vi "motorisedmirrors_coMD.vi"() -> ()   [LabVIEW 2012]
doc: "SciScan 1.2 160622"
uses:
  GFG/GFGstringGet.vi
  <vilib>/Instr/_visa.llb/VISA Configure Serial Port (Instr).vi
  GFG/GFG library.lvlib
panel:
  out "error out":errorcluster
  in  "lock":bool
  in  "SCANHEAD":bool
  in  "MDU":bool
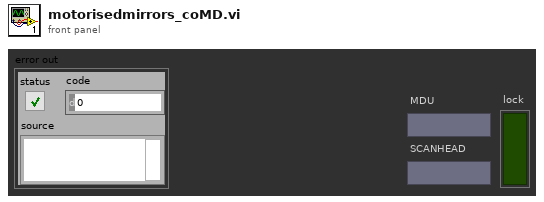
[diagram p1: front panel]
types:
  T1 = enum32{"Invalid", "Standard", "Closed", "Hidden", "Minimized", "Maximized"}
  T2 = enum8{"Enabled", "Disabled", "Disabled and Grayed Out"}
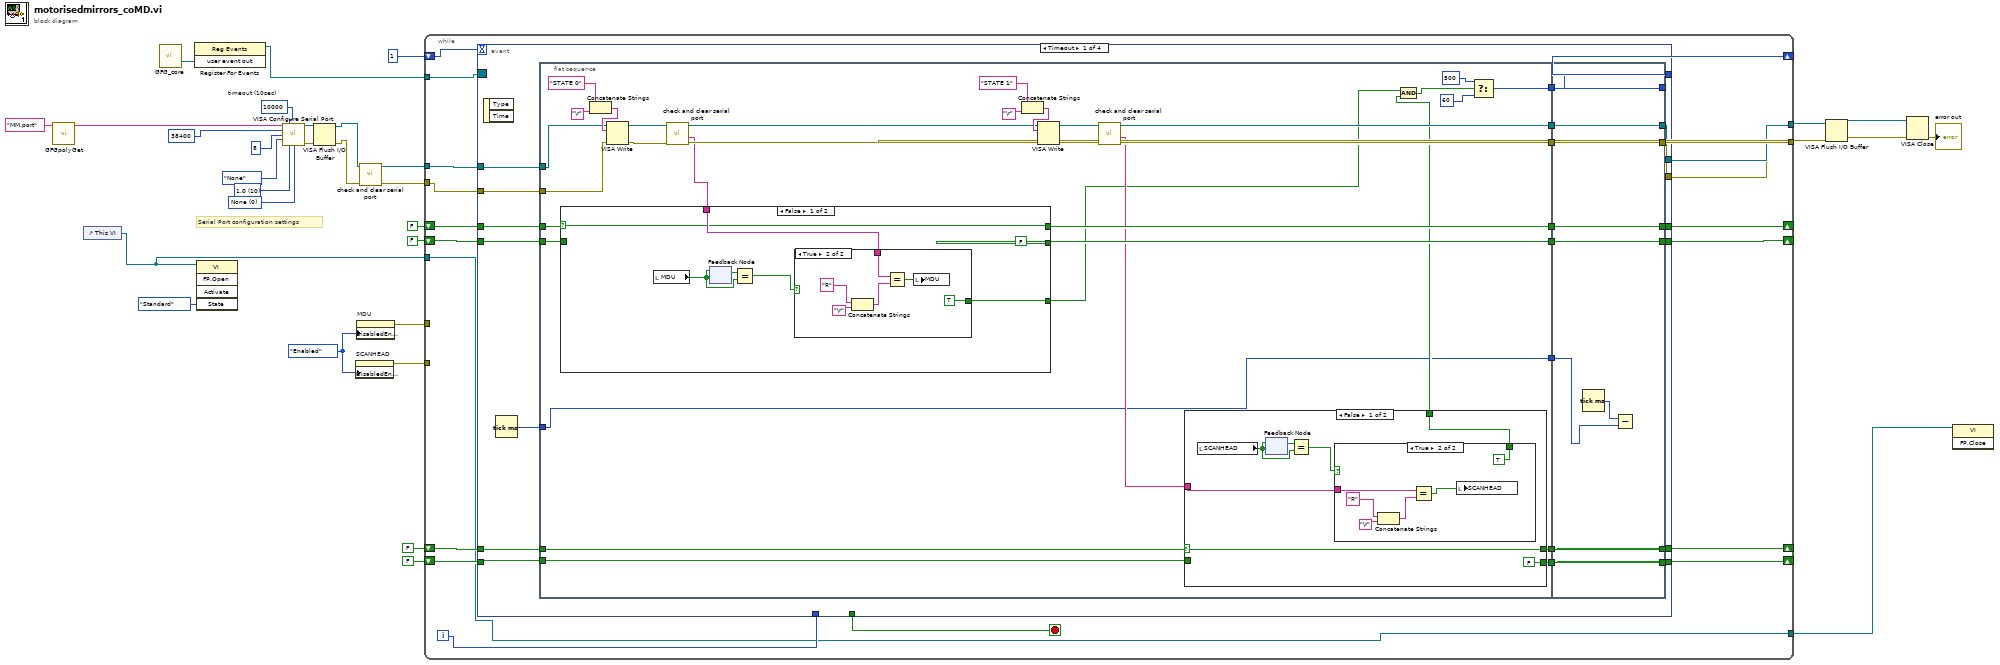
[diagram p0: block diagram]
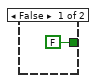
[diagram p2: hidden frame]
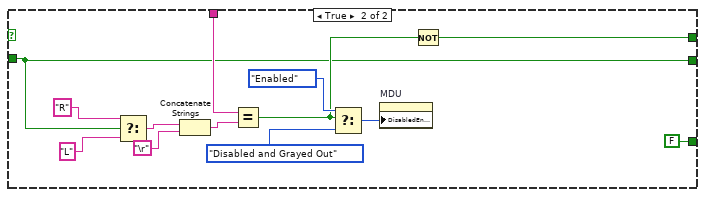
[diagram p3: hidden frame]
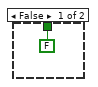
[diagram p4: hidden frame]
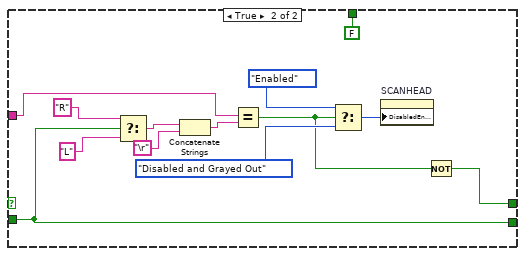
[diagram p5: hidden frame]
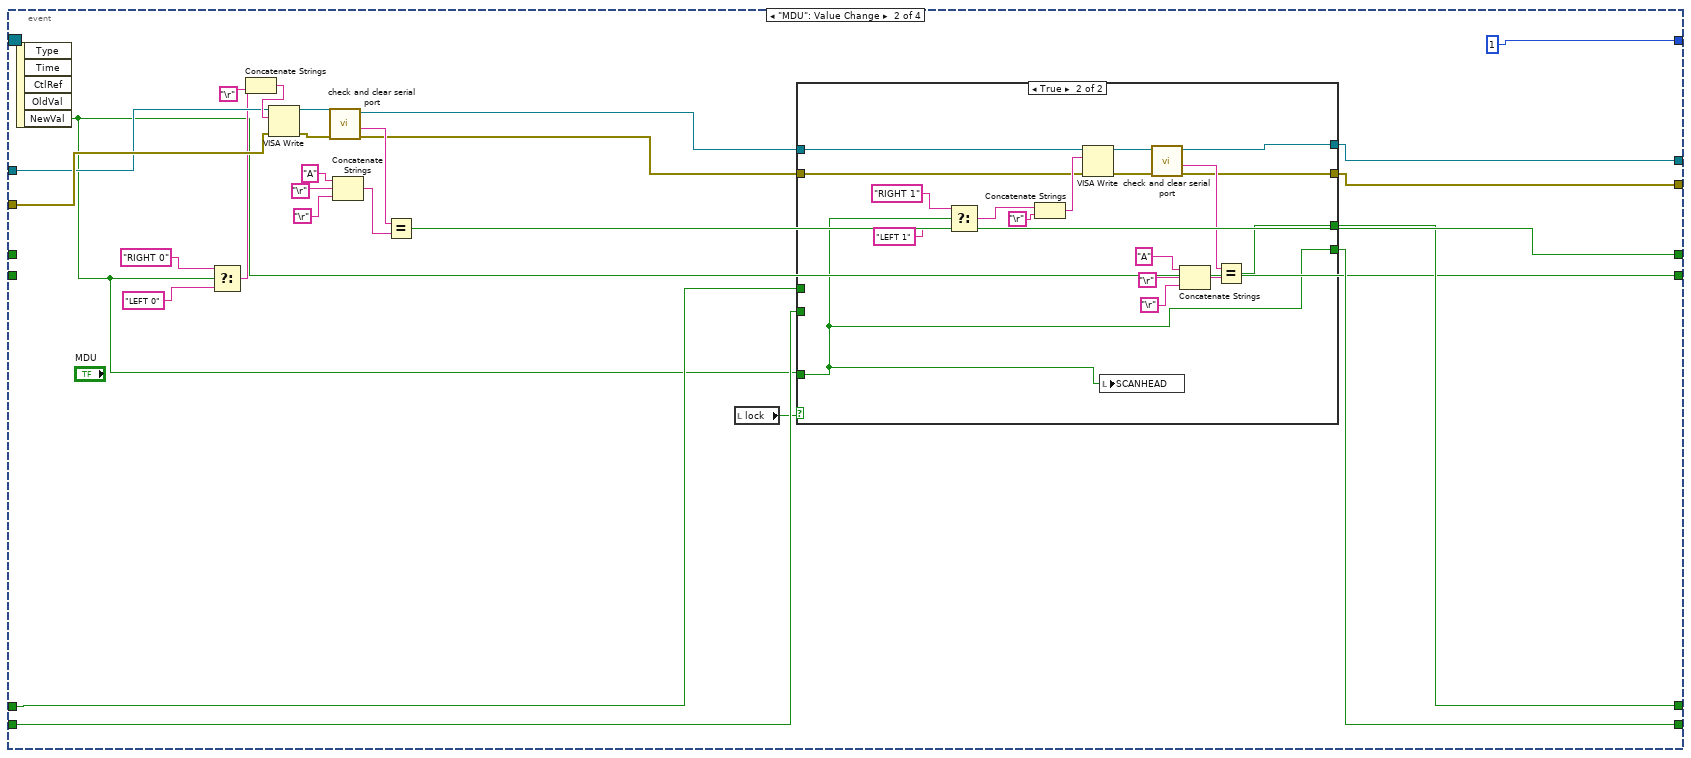
[diagram p6: hidden frame]
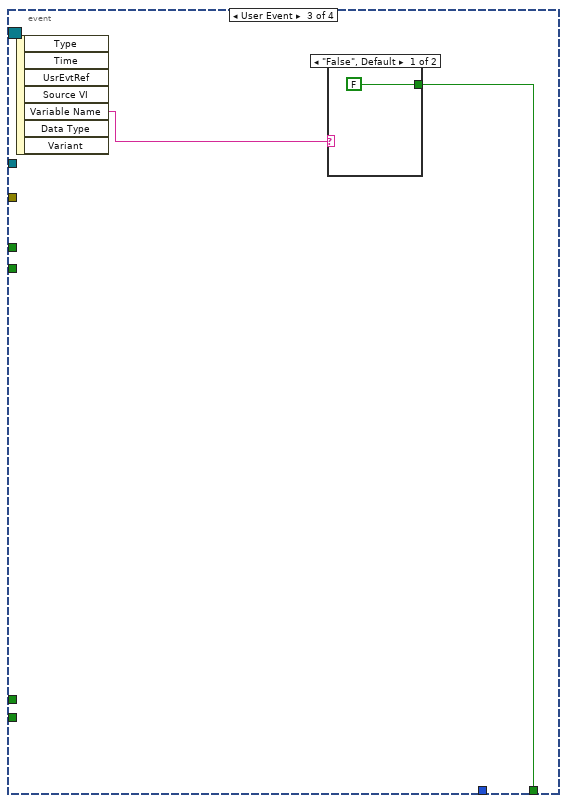
[diagram p8: hidden frame]
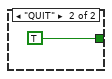
[diagram p9: hidden frame]
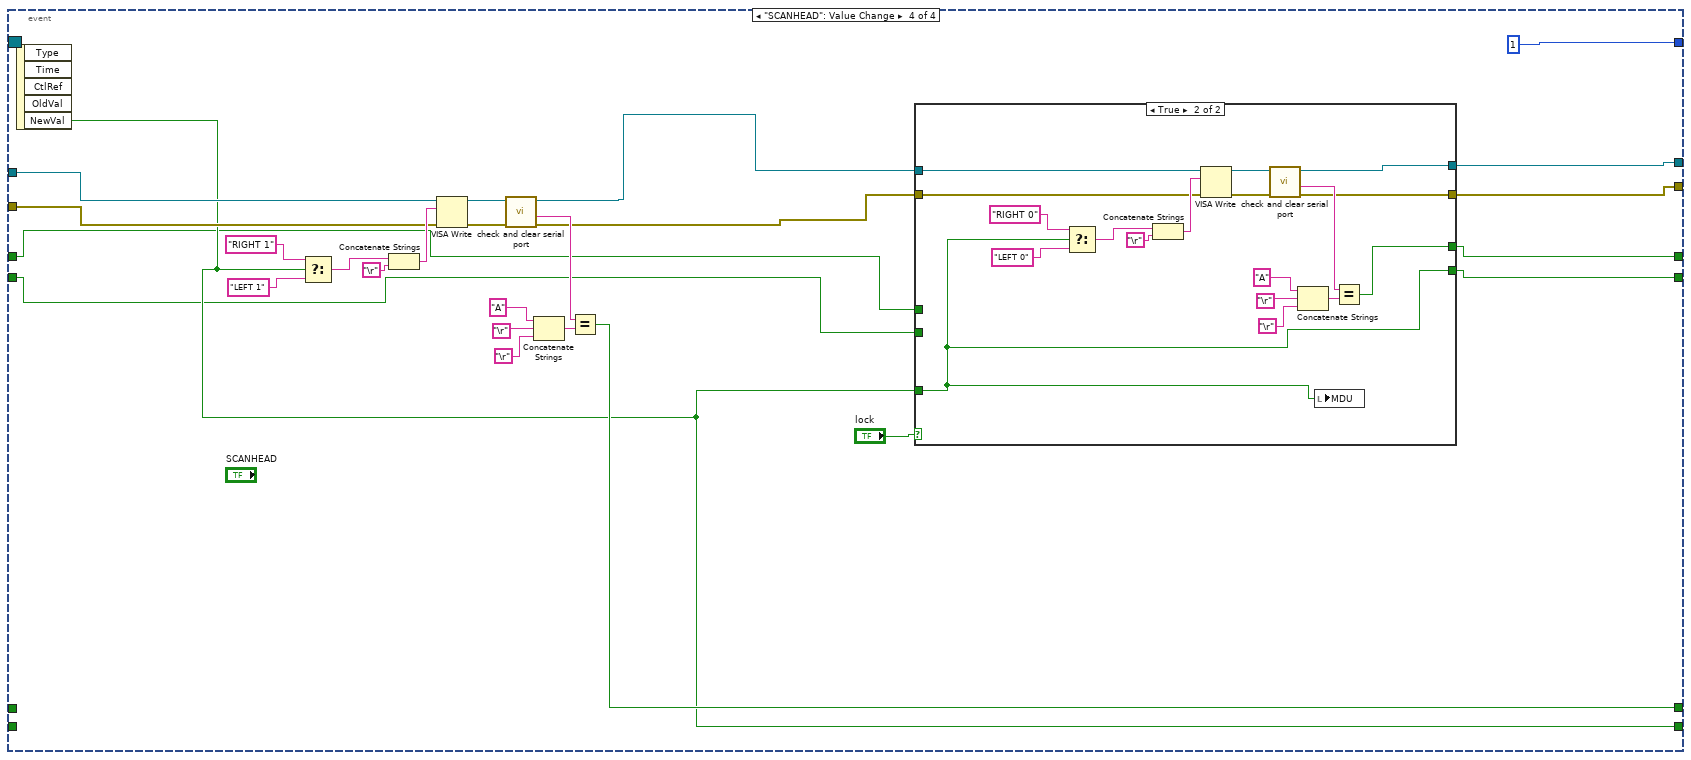
[diagram p10: hidden frame]
diagram:
  w11 = T2."Enabled" ("Disabled")
  w29 = u16 0 items=["None", "XON/XOFF", "RTS/CTS", "XON/XOFF & RTS/CTS", "DTR/DSR", "XON/XOFF & DTR/DSR"] ("flow control (0:none)")
  w28 = u16 10 items=["1.0"=10, "1.5"=15, "2.0"=20] ("stop bits (10: 1 bit)")
  w25 = u32 10000  # timeout (10sec)
  # "Serial Port configuration settings"
  n1 = call-poly "GFGpolyGet.vi"("Variable Name in"="MM.port") -> ("String"=w4:string)  [unwired: 9 in, 1 out]
  n2 = control-ref of="This VI"() -> (w2:refnum<vi>)
  n3 = call "GFG_core.vi"() -> ("user event out"=w8:refnum<user-event>)  [unwired: 13 in, 6 out]
  n4 = register-events(w8) -> (reference out=w7:refnum<event-registration>)  [unwired: 2 in, 1 out]
  n5 = invoke class="VI" method="FP.Open"(reference=w2, "State"=T1."Standard") -> ()  [unwired: 3 in, 5 out]
  n6 = call-poly "VISA Configure Serial Port"("VISA resource name"=w4, "timeout (10sec)"=w25, "baud rate (9600)"=38400, "data bits (8)"=u16 8, "parity (0:none)"=enum16{"None", "Odd", "Even", "Mark", "Space"}."None", "stop bits (10: 1 bit)"=w28, "flow control (0:none)"=w29) -> ("VISA resource name out"=w30:refnum<visa-resource-name>, "error out"=w31:errorcluster)  [unwired: 7 in]
  n7 = VISA Flush I/O Buffer(VISA resource name=w30, error in (no error)=w31) -> (VISA resource name out=w23:refnum<visa-resource-name>, error out=w24:errorcluster)  [unwired: 1 in]
  n8 = property on="SCANHEAD" class="Bool (strict)"("DisabledEnum"=w11) -> (error out=w9:errorcluster)  [unwired: 2 in, 1 out]
  n9 = property on="MDU" class="Bool (strict)"("DisabledEnum"=w11) -> (error out=w10:errorcluster)  [unwired: 2 in, 1 out]
  n10 = call "check and clear serial port.vi"("error in (no error)"=w24, "VISA resource name in"=w23) -> ("error out"=w21:errorcluster, "VISA resource name out"=w22:refnum<visa-resource-name>)  [unwired: 6 in, 2 out]
  n11 = while {
    tunnel: [w50] -> w16
    tunnel: [w49] -> w20
    tunnel: w22 -> [w48]
    tunnel: w21 -> [w47]
    shift-right: [w45] -> _
    shift-left: FALSE -> [w38]
    shift-right: [w43] -> _
    shift-left: 1 -> [w46]
    shift-right: [w42] -> _
    shift-left: FALSE ("MDU") -> [w37]
    shift-right: [w41] -> _
    shift-left: FALSE ("SCANHEAD") -> [w39]
    shift-right: [w44] -> _
    shift-left: FALSE -> [w40]
    tunnel: w10 -> [_]
    tunnel: w9 -> [_]
    tunnel: w7 -> [w35]
    tunnel: w2 -> [w33]
    tunnel: [w33] -> w1
    i -> [w36]
    stop <- w34 stop-if-true
    n12 = event shown="[0] Timeout" {
      selector: w35 -> [_ _ _ _]
      dyn-events: _ -> [_ _ _ _]
      timeout: w46 -> [_ _ _ _]
      tunnel: [w69 w169 _ w229] -> w50
      tunnel: [w70 w176 _ w227] -> w49
      tunnel: w48 -> [w72 w187 _ w240]
      tunnel: w47 -> [w71 w188 _ w241]
      tunnel: [w67 w180 _ w221] -> w45
      tunnel: [w68 w172 _ w231] -> w44
      tunnel: [w64 1 _ 1] -> w43
      tunnel: [w62 w170 _ w222] -> w42
      tunnel: [w60 w173 _ w225] -> w41
      tunnel: w40 -> [w66 w175 _ _]
      tunnel: w39 -> [w61 w174 _ _]
      tunnel: w38 -> [w65 _ _ w224]
      tunnel: w37 -> [w63 _ _ w223]
      tunnel: w36 -> [_ _ _ _]
      tunnel: [_ _ w217 _] -> w34
      event Timeout {
        n13 = event-data() -> ()  [unwired: 1 in, 2 out]
        n14 = Tick Count (ms)() -> (millisecond timer value=w59:u32)
        n15 = flat-sequence {
          tunnel: w72 -> [w103]
          tunnel: w71 -> [w102]
          tunnel: w66 -> [w87]
          tunnel: w65 -> [w86]
          tunnel: w63 -> [w82]
          tunnel: w61 -> [w80]
          tunnel: w59 -> [w73]
          tunnel: [w91] -> w58
          tunnel: [w90] -> w57
          tunnel: [w89] -> w56
          tunnel: [w88] -> w55
          tunnel: [w85] -> w54
          tunnel: [w81] -> w53
          tunnel: [w79] -> w52
          tunnel: [w73] -> w51
          tunnel: [w162] -> w60
          tunnel: [w163] -> w62
          tunnel: [w164] -> w64
          tunnel: [w165] -> w67
          tunnel: [w166] -> w68
          tunnel: [w167] -> w69
          tunnel: [w168] -> w70
          tunnel: w58 -> [w168]
          tunnel: w57 -> [w167]
          tunnel: w56 -> [w166]
          tunnel: w55 -> [w165]
          tunnel: w54 -> [w164]
          tunnel: w53 -> [w163]
          tunnel: w52 -> [w162]
          tunnel: w51 -> [w160]
          frame #0 {
            n16 = Concatenate Strings("STATE 0" ("string"), "\r") -> (w105:string)
            n17 = VISA Write(VISA resource name=w103, write buffer=w105, error in (no error)=w102) -> (VISA resource name out=w95:refnum<visa-resource-name>, error out=w101:errorcluster)  [unwired: 1 out]
            n18 = call "check and clear serial port.vi"("error in (no error)"=w101, "VISA resource name in"=w95) -> ("error out"=w94:errorcluster, "read buffer"=w77:string, "VISA resource name out"=w93:refnum<visa-resource-name>)  [unwired: 6 in, 1 out]
            n19 = case shown="False" w86 {
              selector: w86 -> [w111 _]
              tunnel: w77 -> [w112 w127]
              tunnel: [w111 w123] -> w88
              tunnel: w82 -> [_ w121]
              tunnel: [FALSE ("MDU") w121] -> w81
              tunnel: [w109 FALSE ("SCANHEAD")] -> w76
              frame False {
                n20 = local read "MDU"() -> (w108:bool)
                n21 = feedback #1() -> (w107:bool)  [unwired: 1 in]
                n22 = feedback-in #1(w108) -> ()
                n23 = Equal?(x=w107, y=w108) -> (x = y?=w106:bool)
                n24 = case shown="True" w106 {
                  tunnel: w112 -> [_ w116]
                  tunnel: [FALSE ("SCANHEAD") TRUE ("SCANHEAD")] -> w109
                  frame False {
                  }
                  frame True {
                    n25 = Concatenate Strings("R" ("y"), "\r") -> (w119:string)
                    n26 = Equal?(x=w116, y=w119) -> (x = y?=w115:bool)
                    n27 = local write "MDU"(w115) -> ()
                  }
                }
              }
              frame True {
                n28 = Select(t="R" ("string"), s=w121, f="L" ("string")) -> (s? t:f=w129:string)
                n29 = Concatenate Strings(w129, "\r") -> (w132:string)
                n30 = Equal?(x=w127, y=w132) -> (x = y?=w124:bool)
                n31 = Select(t=T2."Enabled" ("Disabled"), s=w124, f=T2."Disabled and Grayed Out" ("Disabled")) -> (s? t:f=w122:T2)
                n32 = property on="MDU" class="Bool (strict)"("DisabledEnum"=w122) -> ()  [unwired: 2 in, 2 out]
                n33 = Not(x=w124) -> (.not. x?=w123:bool)
              }
            }
            n34 = Concatenate Strings("STATE 1" ("string"), "\r") -> (w96:string)
            n35 = VISA Write(VISA resource name=w93, write buffer=w96, error in (no error)=w94) -> (VISA resource name out=w92:refnum<visa-resource-name>, error out=w98:errorcluster)  [unwired: 1 out]
            n36 = call "check and clear serial port.vi"("error in (no error)"=w98, "VISA resource name in"=w92) -> ("error out"=w91:errorcluster, "read buffer"=w78:string, "VISA resource name out"=w90:refnum<visa-resource-name>)  [unwired: 6 in, 1 out]
            n37 = case shown="False" w87 {
              selector: w87 -> [w138 _]
              tunnel: w78 -> [w139 w154]
              tunnel: [w138 w149] -> w89
              tunnel: w80 -> [_ w148]
              tunnel: [FALSE ("SCANHEAD") w148] -> w79
              tunnel: [w136 FALSE ("SCANHEAD")] -> w75
              frame False {
                n38 = local read "SCANHEAD"() -> (w134:bool)
                n39 = feedback #2() -> (w135:bool)  [unwired: 1 in]
                n40 = feedback-in #2(w134) -> ()
                n41 = Equal?(x=w135, y=w134) -> (x = y?=w133:bool)
                n42 = case shown="True" w133 {
                  tunnel: w139 -> [_ w143]
                  tunnel: [FALSE ("SCANHEAD") TRUE ("SCANHEAD")] -> w136
                  frame False {
                  }
                  frame True {
                    n43 = Concatenate Strings("R" ("y"), "\r") -> (w146:string)
                    n44 = Equal?(x=w143, y=w146) -> (x = y?=w142:bool)
                    n45 = local write "SCANHEAD"(w142) -> ()
                  }
                }
              }
              frame True {
                n46 = Select(t="R" ("string"), s=w148, f="L" ("string")) -> (s? t:f=w156:string)
                n47 = Concatenate Strings(w156, "\r") -> (w159:string)
                n48 = Equal?(x=w154, y=w159) -> (x = y?=w150:bool)
                n49 = Select(t=T2."Enabled" ("Disabled"), s=w150, f=T2."Disabled and Grayed Out" ("Disabled")) -> (s? t:f=w151:T2)
                n50 = property on="SCANHEAD" class="Bool (strict)"("DisabledEnum"=w151) -> ()  [unwired: 2 in, 2 out]
                n51 = Not(x=w150) -> (.not. x?=w149:bool)
              }
            }
            n52 = And(x=w76, y=w75) -> (x .and. y?=w74:bool)
            n53 = Select(t=500, s=w74, f=60) -> (s? t:f=w85:i32)
          }
          frame #1 {
            n54 = Tick Count (ms)() -> (millisecond timer value=w161:u32)
            n55 = Subtract(x=w161, y=w160) -> ()  [unwired: 1 out]
          }
        }
      }
      event "MDU": Value Change {
        n56 = event-data() -> ("NewVal"=w170:bool)  [unwired: 1 in, 4 out]
        n57 = Select(t="RIGHT 0" ("write buffer"), s=w170, f="LEFT 0" ("write buffer 2")) -> (s? t:f=w186:string)
        n58 = Concatenate Strings(w186, "\r") -> (w192:string)
        n59 = VISA Write(VISA resource name=w187, write buffer=w192, error in (no error)=w188) -> (VISA resource name out=w189:refnum<visa-resource-name>, error out=w190:errorcluster)  [unwired: 1 out]
        n60 = call "check and clear serial port.vi"("error in (no error)"=w190, "VISA resource name in"=w189) -> ("error out"=w177:errorcluster, "read buffer"=w183:string, "VISA resource name out"=w178:refnum<visa-resource-name>)  [unwired: 6 in, 1 out]
        n61 = Concatenate Strings("A" ("string"), "\r", "\r") -> (w182:string)
        n62 = Equal?(x=w183, y=w182) -> (x = y?=w180:bool)
        n63 = local read "lock"() -> (w171:bool)
        n64 = case shown="True" w171 {
          tunnel: w178 -> [w197 w204]
          tunnel: [w197 w203] -> w169
          tunnel: w177 -> [w198 w202]
          tunnel: [w198 w201] -> w176
          tunnel: w170 -> [_ w199]
          tunnel: w175 -> [w196 _]
          tunnel: w174 -> [w195 _]
          tunnel: [w196 w200] -> w172
          tunnel: [w195 w199] -> w173
          frame False {
          }
          frame True {
            n65 = Select(t="RIGHT 1" ("write buffer"), s=w199, f="LEFT 1" ("write buffer 2")) -> (s? t:f=w213:string)
            n66 = Concatenate Strings(w213, "\r") -> (w216:string)
            n67 = VISA Write(VISA resource name=w204, write buffer=w216, error in (no error)=w202) -> (VISA resource name out=w211:refnum<visa-resource-name>, error out=w210:errorcluster)  [unwired: 1 out]
            n68 = local write "SCANHEAD"(w199) -> ()
            n69 = call "check and clear serial port.vi"("error in (no error)"=w210, "VISA resource name in"=w211) -> ("error out"=w201:errorcluster, "read buffer"=w205:string, "VISA resource name out"=w203:refnum<visa-resource-name>)  [unwired: 6 in, 1 out]
            n70 = Concatenate Strings("A" ("string"), "\r", "\r") -> (w206:string)
            n71 = Equal?(x=w205, y=w206) -> (x = y?=w200:bool)
          }
        }
      }
      event User Event {
        n72 = event-data() -> ("Variable Name"=w218:string)  [unwired: 1 in, 6 out]
        n73 = case shown="\"False\", Default" w218 {
          tunnel: [FALSE TRUE] -> w217
          frame "False", Default {
          }
          frame "QUIT" {
          }
        }
      }
      event "SCANHEAD": Value Change {
        n74 = event-data() -> ("NewVal"=w225:bool)  [unwired: 1 in, 4 out]
        n75 = Select(t="RIGHT 1" ("write buffer"), s=w225, f="LEFT 1" ("write buffer 2")) -> (s? t:f=w243:string)
        n76 = Concatenate Strings(w243, "\r") -> (w246:string)
        n77 = VISA Write(VISA resource name=w240, write buffer=w246, error in (no error)=w241) -> (VISA resource name out=w239:refnum<visa-resource-name>, error out=w238:errorcluster)  [unwired: 1 out]
        n78 = call "check and clear serial port.vi"("error in (no error)"=w238, "VISA resource name in"=w239) -> ("error out"=w228:errorcluster, "read buffer"=w232:string, "VISA resource name out"=w230:refnum<visa-resource-name>)  [unwired: 6 in, 1 out]
        n79 = Concatenate Strings("A" ("string"), "\r", "\r") -> (w234:string)
        n80 = Equal?(x=w232, y=w234) -> (x = y?=w231:bool)
        n81 = case shown="True" "lock" {
          tunnel: w230 -> [w249 w256]
          tunnel: [w249 w255] -> w229
          tunnel: w228 -> [w250 w254]
          tunnel: [w250 w253] -> w227
          tunnel: w225 -> [_ w251]
          tunnel: w224 -> [w248 _]
          tunnel: w223 -> [w247 _]
          tunnel: [w248 w252] -> w221
          tunnel: [w247 w251] -> w222
          frame False {
          }
          frame True {
            n82 = Select(t="RIGHT 0" ("write buffer"), s=w251, f="LEFT 0" ("write buffer 2")) -> (s? t:f=w265:string)
            n83 = Concatenate Strings(w265, "\r") -> (w268:string)
            n84 = VISA Write(VISA resource name=w256, write buffer=w268, error in (no error)=w254) -> (VISA resource name out=w263:refnum<visa-resource-name>, error out=w262:errorcluster)  [unwired: 1 out]
            n85 = call "check and clear serial port.vi"("error in (no error)"=w262, "VISA resource name in"=w263) -> ("error out"=w253:errorcluster, "read buffer"=w257:string, "VISA resource name out"=w255:refnum<visa-resource-name>)  [unwired: 6 in, 1 out]
            n86 = Concatenate Strings("A" ("string"), "\r", "\r") -> (w258:string)
            n87 = local write "MDU"(w251) -> ()
            n88 = Equal?(x=w257, y=w258) -> (x = y?=w252:bool)
          }
        }
      }
    }
  }
  n89 = VISA Flush I/O Buffer(VISA resource name=w16, error in (no error)=w20) -> (VISA resource name out=w18:refnum<visa-resource-name>, error out=w19:errorcluster)  [unwired: 1 in]
  n90 = VISA Close(VISA resource name=w18, error in (no error)=w19) -> (error out=→"error out":errorcluster)
  n91 = invoke class="VI" method="FP.Close"(reference=w1) -> ()  [unwired: 2 in, 3 out]
